vi "流程写入仪器.vi"(7 "流程":u16[](array[numeric]) format="%04xH", 8 "error in (no error)":errorcluster, 9 "量程":enum16{"低量程", "高量程"}(ring), 10 "测量模式":enum16{"跨度核查", "水样测量", "零点核查", "标样核查", "加标回收"}(ring), 11 "参数":u16(ring) items=["总磷"=1, "总氮"=2, "氨氮"=3]) -> (0 "error out":errorcluster, 2 "步数":i32, 3 "参数编码":u16[](array[numeric]) format="%04xH")   [LabVIEW 2016, in "斯坦道总磷总氮V2.lvlib"]
uses:
  <vilib>/Plasmionique/MB Master/MB Master.lvlib
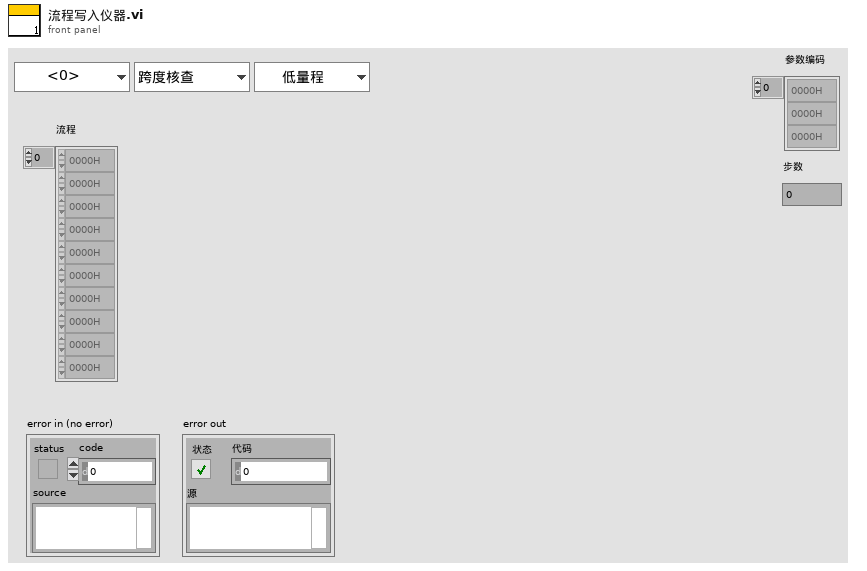
[diagram p1: front panel]
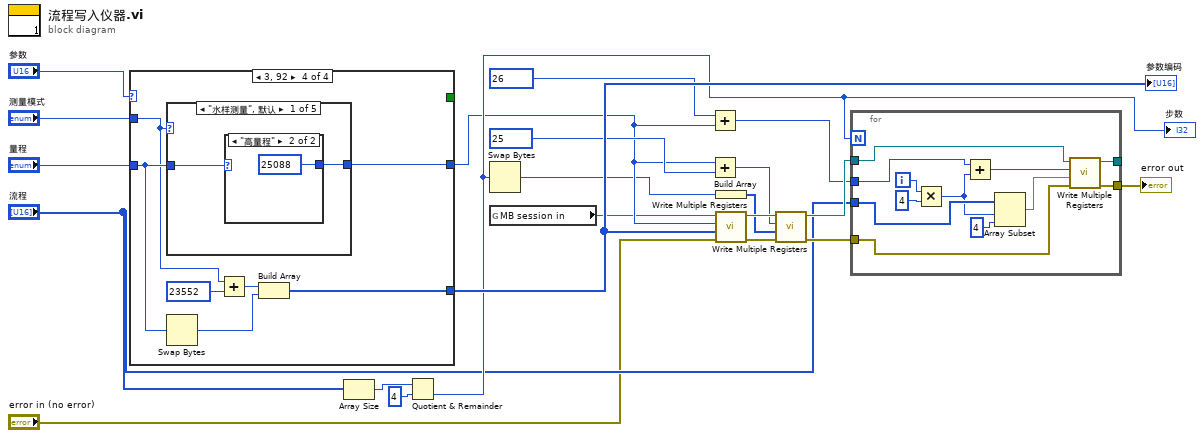
[diagram p0: block diagram]
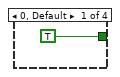
[diagram p2: hidden frame]
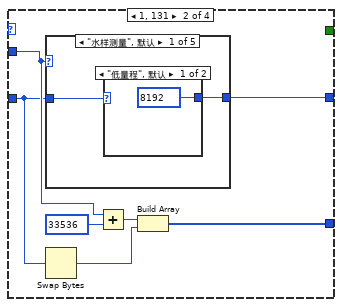
[diagram p3: hidden frame]
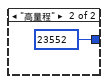
[diagram p4: hidden frame]
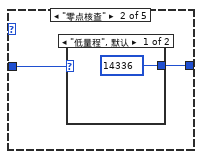
[diagram p5: hidden frame]
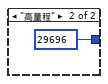
[diagram p6: hidden frame]
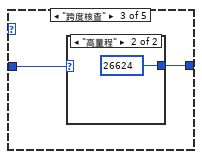
[diagram p7: hidden frame]
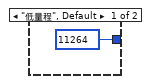
[diagram p8: hidden frame]
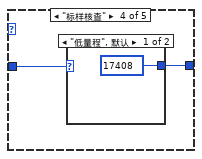
[diagram p9: hidden frame]
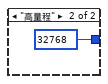
[diagram p10: hidden frame]
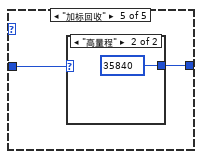
[diagram p11: hidden frame]
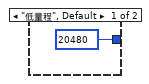
[diagram p12: hidden frame]
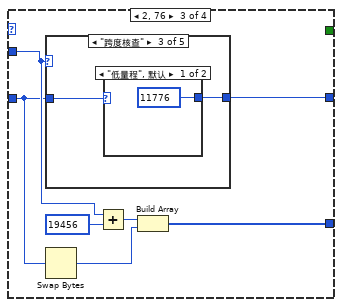
[diagram p13: hidden frame]
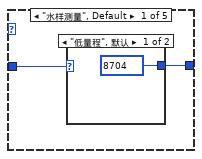
[diagram p14: hidden frame]
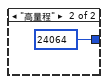
[diagram p15: hidden frame]
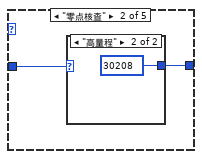
[diagram p16: hidden frame]
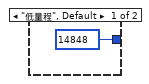
[diagram p17: hidden frame]
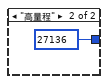
[diagram p18: hidden frame]
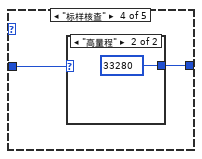
[diagram p19: hidden frame]
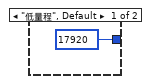
[diagram p20: hidden frame]
diagram:
  n1 = case shown="3, 92" "参数" {
    tunnel: "测量模式" -> [_ w28 w53 w79]
    tunnel: "量程" -> [_ w27 w52 w80]
    tunnel: [_ w30 w57 w84] -> w8
    tunnel: [TRUE _ _ _] -> _
    tunnel: [_ w24 w51 w78] -> w17
    frame 0, Default {
    }
    frame 1, 131 {
      n2 = case shown="\"水样测量\", 默认" w28 {
        tunnel: w27 -> [w32 w36 w40 w44 w48]
        tunnel: [w31 w35 w39 w43 w47] -> w30
        frame "水样测量", Default {
          n3 = case shown="\"低量程\", 默认" w32 {
            tunnel: [u16 8192 ("starting address") u16 23552 ("starting address")] -> w31
            frame "低量程", Default {
            }
            frame "高量程" {
            }
          }
        }
        frame "零点核查" {
          n4 = case shown="\"低量程\", 默认" w36 {
            tunnel: [u16 14336 ("starting address") u16 29696 ("starting address")] -> w35
            frame "低量程", Default {
            }
            frame "高量程" {
            }
          }
        }
        frame "跨度核查" {
          n5 = case shown="\"高量程\"" w40 {
            tunnel: [u16 11264 ("starting address") u16 26624 ("starting address")] -> w39
            frame "低量程", Default {
            }
            frame "高量程" {
            }
          }
        }
        frame "标样核查" {
          n6 = case shown="\"低量程\", 默认" w44 {
            tunnel: [u16 17408 ("starting address") u16 32768 ("starting address")] -> w43
            frame "低量程", Default {
            }
            frame "高量程" {
            }
          }
        }
        frame "加标回收" {
          n7 = case shown="\"高量程\"" w48 {
            tunnel: [u16 20480 ("starting address") u16 35840 ("starting address")] -> w47
            frame "低量程", Default {
            }
            frame "高量程" {
            }
          }
        }
      }
      n8 = Swap Bytes(anything=w27) -> (byte swapped=w26:u16)
      n9 = Add(x=w28, y=u16 33536 ("starting address")) -> (x+y=w25:u16)
      n10 = Build Array(w25, w26) -> (w24:u16[])
    }
    frame 2, 76 {
      n11 = case shown="\"跨度核查\"" w53 {
        tunnel: w52 -> [w59 w63 w67 w71 w75]
        tunnel: [w58 w62 w66 w70 w74] -> w57
        frame "水样测量", Default {
          n12 = case shown="\"低量程\", 默认" w59 {
            tunnel: [u16 8704 ("starting address") u16 24064 ("starting address")] -> w58
            frame "低量程", Default {
            }
            frame "高量程" {
            }
          }
        }
        frame "零点核查" {
          n13 = case shown="\"高量程\"" w63 {
            tunnel: [u16 14848 ("starting address") u16 30208 ("starting address")] -> w62
            frame "低量程", Default {
            }
            frame "高量程" {
            }
          }
        }
        frame "跨度核查" {
          n14 = case shown="\"低量程\", 默认" w67 {
            tunnel: [u16 11776 ("starting address") u16 27136 ("starting address")] -> w66
            frame "低量程", Default {
            }
            frame "高量程" {
            }
          }
        }
        frame "标样核查" {
          n15 = case shown="\"高量程\"" w71 {
            tunnel: [u16 17920 ("starting address") u16 33280 ("starting address")] -> w70
            frame "低量程", Default {
            }
            frame "高量程" {
            }
          }
        }
        frame "加标回收" {
          n16 = case shown="\"低量程\", 默认" w75 {
            tunnel: [u16 20992 ("starting address") u16 36352 ("starting address")] -> w74
            frame "低量程", Default {
            }
            frame "高量程" {
            }
          }
        }
      }
      n17 = Swap Bytes(anything=w52) -> (byte swapped=w55:u16)
      n18 = Add(x=w53, y=u16 19456 ("starting address")) -> (x+y=w54:u16)
      n19 = Build Array(w54, w55) -> (w51:u16[])
    }
    frame 3, 92 {
      n20 = case shown="\"水样测量\", 默认" w79 {
        tunnel: w80 -> [w86 w90 w94 w98 w102]
        tunnel: [w85 w89 w93 w97 w101] -> w84
        frame "水样测量", Default {
          n21 = case shown="\"高量程\"" w86 {
            tunnel: [u16 9728 ("starting address") u16 25088 ("starting address")] -> w85
            frame "低量程", Default {
            }
            frame "高量程" {
            }
          }
        }
        frame "零点核查" {
          n22 = case shown="\"低量程\", 默认" w90 {
            tunnel: [u16 15872 ("starting address") u16 31232 ("starting address")] -> w89
            frame "低量程", Default {
            }
            frame "高量程" {
            }
          }
        }
        frame "跨度核查" {
          n23 = case shown="\"低量程\", 默认" w94 {
            tunnel: [u16 12800 ("starting address") u16 28160 ("starting address")] -> w93
            frame "低量程", Default {
            }
            frame "高量程" {
            }
          }
        }
        frame "标样核查" {
          n24 = case shown="\"高量程\"" w98 {
            tunnel: [u16 18944 ("starting address") u16 34304 ("starting address")] -> w97
            frame "低量程", Default {
            }
            frame "高量程" {
            }
          }
        }
        frame "加标回收" {
          n25 = case shown="\"低量程\", 默认" w102 {
            tunnel: [u16 22016 ("starting address") u16 37376 ("starting address")] -> w101
            frame "低量程", Default {
            }
            frame "高量程" {
            }
          }
        }
      }
      n26 = Swap Bytes(anything=w80) -> (byte swapped=w82:u16)
      n27 = Add(x=w79, y=u16 23552 ("starting address")) -> (x+y=w81:u16)
      n28 = Build Array(w81, w82) -> (w78:u16[])
    }
  }
  "参数编码" <- w17
  n29 = Array Size(array="流程") -> (size(s)=w19:i32)
  n30 = Quotient & Remainder(x=w19, y=u16 4) -> (floor(x/y)=w12:i32)  [unwired: 1 out]
  "步数" <- w12
  n31 = Swap Bytes(anything=w12) -> (byte swapped=w1:i32)
  n32 = global read "VAR总磷总氮全局变量.vi" "MB session in"() -> (w4:refnum<class "MB_Master.lvclass">)
  n33 = Add(x=u16 26 ("starting address"), y=w8) -> (x+y=w6:u16)
  n34 = Add(x=w8, y=u16 25 ("starting address")) -> (x+y=w13:u16)
  n35 = Build Array(w1) -> (w11:i32[])
  n36 = call <vilib>:"Write Multiple Registers.vi"("error in (no error)"="error in (no error)", "values"=w17, "starting address"=w8, "MB session in"=w4) -> ("error out"=w15:errorcluster, "MB session out"=w16:refnum<class "MB_Master.lvclass">)  [unwired: 6 in]
  n37 = call <vilib>:"Write Multiple Registers.vi"("error in (no error)"=w15, "values"=w11, "starting address"=w13, "MB session in"=w16) -> ("error out"=w9:errorcluster, "MB session out"=w10:refnum<class "MB_Master.lvclass">)  [unwired: 6 in]
  n38 = for {
    N: w12 -> [_]
    tunnel: "流程" -> [w114]
    tunnel: w10 -> [w116]
    tunnel: w9 -> [w115]
    tunnel: w6 -> [w112]
    tunnel: [w108] -> _
    tunnel: [w107] -> w2
    i -> [w111]
    n39 = Multiply(x=w111, y=4) -> (x*y=w105:i32)
    n40 = Add(x=w112, y=w105) -> (x+y=w109:i32)
    n41 = Array Subset(array=w114, index=w105, length=4 ("长度")) -> (w106:u16[])
    n42 = call <vilib>:"Write Multiple Registers.vi"("error in (no error)"=w115, "values"=w106, "starting address"=w109, "MB session in"=w116) -> ("error out"=w107:errorcluster, "MB session out"=w108:refnum<class "MB_Master.lvclass">)  [unwired: 6 in]
  }
  "error out" <- w2
